vi "Insert-header.vi"(10 "Header 2":string, 11 "Header 1":string) -> (3 "concatenated string":string)   [LabVIEW 2014]
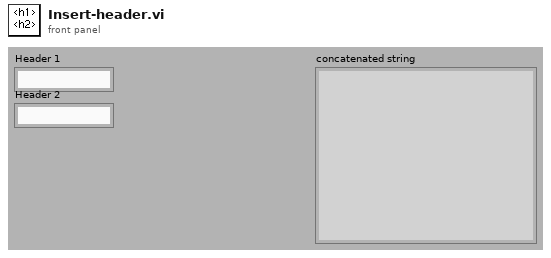
[diagram p1: front panel]
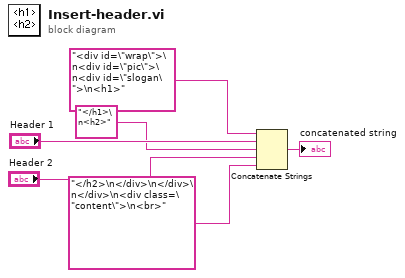
[diagram p0: block diagram]
diagram:
  n1 = Concatenate Strings("<div id=\"wrap\">\n<div id=\"pic\">\n<div id=\"slogan\">\n<h1>" ("HTML"), "Header 1", "</h1>\n<h2>" ("HTML"), "Header 2", "</h2>\n</div>\n</div>\n</div>\n<div class=\"content\">\n<br>" ("HTML")) -> (→"concatenated string":string)
